vi "ChkElekExist.vi"(1 "Data":string[][](array[string]), 2 "Floor":string) -> (0 "布尔":bool)   [LabVIEW 2012]
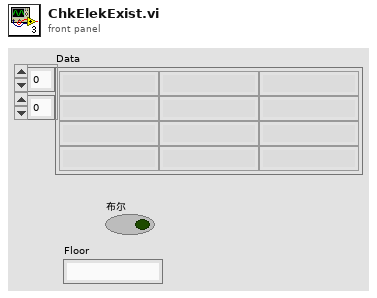
[diagram p1: front panel]
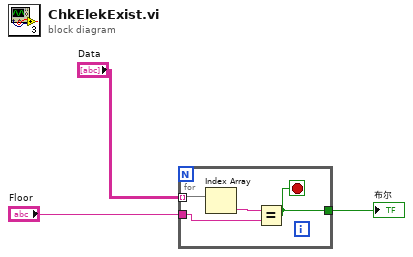
[diagram p0: block diagram]
diagram:
  n1 = for {
    tunnel: "Data" -> [w7] mode=indexing
    tunnel: "Floor" -> [w4]
    tunnel: [w5] -> w3
    stop <- w5 stop-if-true
    n2 = Index Array(array=w7) -> (element=w6:string)  [unwired: 1 in]
    n3 = Equal?(x=w6, y=w4) -> (x = y?=w5:bool)
  }
  "布尔" <- w3
